vi "Launch Fault Monitor.vi"(8 "error in":errorcluster, 11 "Base Software in":refnum<class "Base Software.lvclass">) -> (0 "error out":errorcluster, 3 "Base Software out":refnum<class "Base Software.lvclass">)   [LabVIEW 2019, in "Base Software.lvlib" / "Main.lvlib" / "Base Software.lvclass"]
uses:
  Project/Base Software.lvclass
  builds/Base Software/Panels/Fault Handler.lvlibp/Project/Fault Handler.lvclass
  C:/Users/Public/Documents/Development/builds/Engine/Engine.lvlibp/Project/Engine.lvclass
  builds/Engine/Panel Manager.lvlibp/Panel Actor/Panel Actor.lvclass
  builds/Engine/Panel.lvlibp/Panel/Panel.lvclass
  Custom Controls/Panel_Positions.ctl
  builds/Engine/Panel.lvlibp/Panel/Subpanel/Subpanel.lvclass
  C:/Users/Public/Documents/Development/builds/Engine/Panel.lvlibp/Panel/Panel.lvclass
  builds/Engine/Engine.lvlibp/Project/Engine.lvclass
  C:/Users/Public/Documents/Development/builds/Engine/Panel Manager.lvlibp/Panel Actor/Panel Actor.lvclass
  Accessors/GUI/Read Bottom Panel ref.vi
  builds/Engine/Panel.lvlibp/Panel/Subpanel/Subpanel.vi
  Custom Controls/g_Identifiers.vi
  builds/Engine/Panel.lvlibp
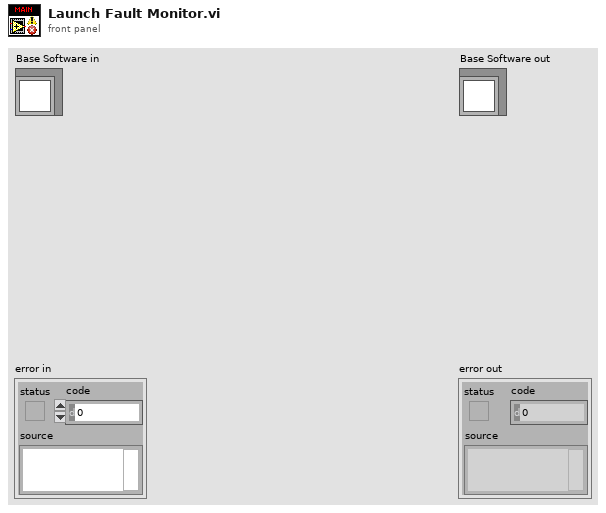
[diagram p1: front panel]
types:
  T1 = typedef "Base Software.lvlib/Main.lvlib/Base Software.lvclass/Panel_Positions.ctl" = enum16{"Prime", "Right", "Bottom", "Left", "Mission"}
  T2 = cluster{"Panel Actor":refnum<class "Panel Actor.lvclass">, "Panel":refnum<class "Panel.lvclass">}
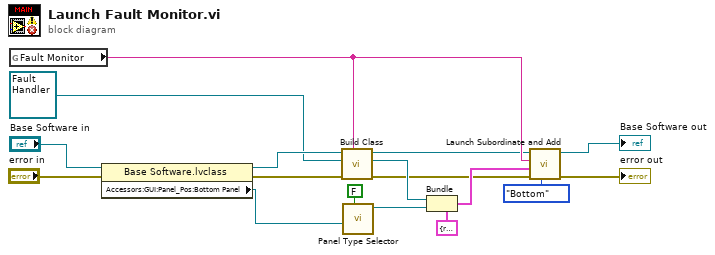
[diagram p0: block diagram]
diagram:
  n1 = global read "g_Identifiers.vi" "Fault Monitor"() -> (w8:string)
  n2 = property class="Base Software.lvclass"(reference="Base Software in", error in="error in") -> (reference out=w9:refnum<class "Base Software.lvclass">, error out=w4:errorcluster, "Accessors:GUI:Panel_Pos:Bottom Panel"=w11:refnum<vi>)
  n3 = call-dynamic "Build Class.vi"("Actor Label"=w8, "error in (no error)"=w4, "Actor in"=refnum<class "Fault Handler.lvclass"> refnum ("Fault Handler.lvlibp:Fault Handler.lvclass"), "Engine in"=w9) -> ("error out"=w3:errorcluster, "Actor out"=w5:refnum<class "Engine.lvclass">, "Engine out"=w7:refnum<class "Base Software.lvclass">)  [unwired: 5 in]
  n4 = call-poly "Panel Type Selector.vi"("Autoshow? (T)"=FALSE, "Sub Panel"=w11) -> ("Subpanel Out"=w15:refnum<class "Subpanel.lvclass">)  [unwired: 8 in, 1 out]
  n5 = Bundle(cluster=T2 {"Panel Actor"=refnum, "Panel"=refnum} ("Panel Definiton"), "Panel Actor"=w5, "Panel"=w15) -> (w14:T2)
  n6 = call "Launch Subordinate and Add.vi"("Position"=Panel_Positions."Bottom", "error in"=w3, "Panel Definiton"=w14, "Identifier"=w8, "Base Software in"=w7) -> ("error out"=→"error out":errorcluster, "Base Software out"=→"Base Software out":refnum<class "Base Software.lvclass">)  [unwired: 5 in]
